vi "nelder_sort.vi"(11 "input simplex":sgl[][](array[numeric])) -> (3 "output simplex":sgl[][](array[numeric]))   [LabVIEW 2018]
uses:
  d4327ab3-bf3d-4415-8528-64425b870461.vi
  <vilib>/Array/Sort 2D Array - Pop Stack.vi
  <vilib>/Array/Sort 2D Array - Push Stack.vi
  d4327ab3-bf3d-4415-8528-64425b870461.vi/4c8b5367-eb1a-476a-b90a-6df11962efe5.vi
  d4327ab3-bf3d-4415-8528-64425b870461.vi/1f408b82-1a71-4455-9f10-7ac211076656.vi
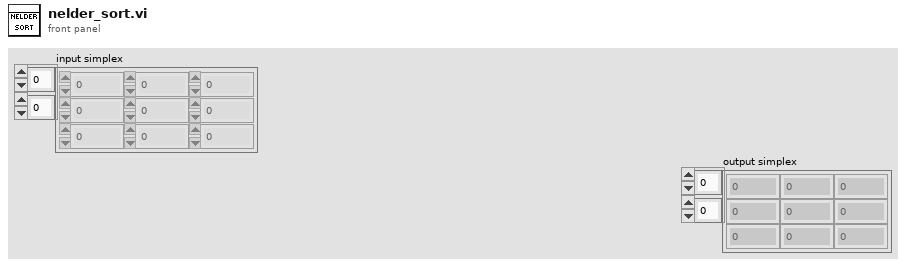
[diagram p1: front panel]
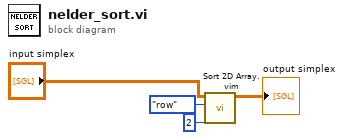
[diagram p0: block diagram]
diagram:
  n1 = call "Sort 2D Array.vim"("index"=2, "dimension to index (column)"=enum16{"column", "row"}."row", "2D array"="input simplex") -> ("sorted 2D array"=→"output simplex":sgl[][])  [unwired: 7 in, 1 out]
